vi "FIR Windowed Coefficients.vi"(0 "filter type":T2, 1 "high cutoff freq: fh":dbl=0.45 format="%0.2f", 2 "window parameter":dbl=nan, 5 "sampling freq: fs":dbl=1.0 format="%0.2f", 7 "taps":i32=25 min=1, 9 "window":T1 items=["Rectangle"=0, "Hanning"=1, "Hamming"=2, "Blackman-Harris"=3, "Exact Blackman"=4, "Blackman"=5, "Flat Top"=6, "4 Term B-Harris "=7, "7 Term B-Harris"=8, "Low Sidelobe"=9, "Blackman Nuttall"=11, "Triangle"=30, "Bartlett-Hanning"=31, "Bohman"=32, "Parzen"=33, "Welch"=34, "Kaiser"=60, "Dolph-Chebyshev"=61, "Gaussian"=62], 11 "option":enum32{"not scaled", "scaled"}(ring), 12 "low cutoff freq: fl":dbl=0.125 format="%0.2f") -> (4 "FIR Windowed Coefficients":dbl[](array[numeric]), 15 "error":i32)   [LabVIEW 2017, in "NI_AALBase.lvlib"]
doc: "Generates the set of filter coefficients you need to implement an FIR windowed filter."
uses:
  <vilib>/Analysis/NI_AALBase.lvlib
  <vilib>/Analysis/3filter.llb/Filter Passband Type.ctl
  <vilib>/Analysis/4window.llb/windowTd.ctl
  <vilib>/Analysis/1siggen.llb/Ramp Pattern by Samples.vi
  <vilib>/Analysis/4window.llb/Symmetric Window (DBL).vi
  <vilib>/Analysis/NI_AALPro.lvlib
panel:
  # "FIR Windowed Filter Coefficients"
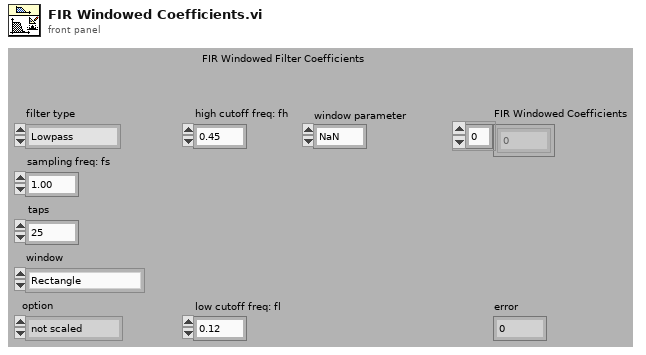
[diagram p1: front panel]
types:
  T1 = typedef "NI_AALPro.lvlib/windowTd.ctl" = u32
  T2 = typedef "NI_AALBase.lvlib/Filter Passband Type.ctl" = enum32{"Lowpass", "Highpass", "Bandpass", "Bandstop"}
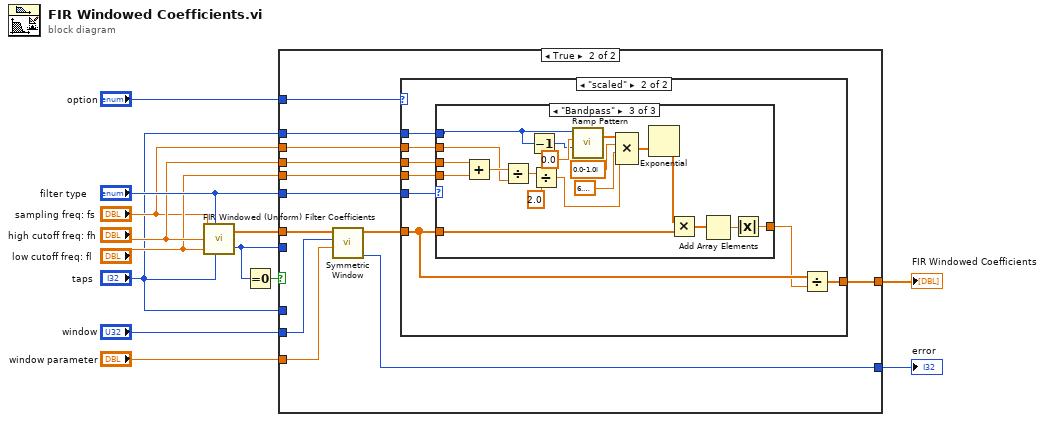
[diagram p0: block diagram]
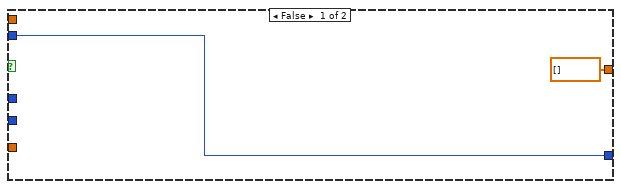
[diagram p2: hidden frame]
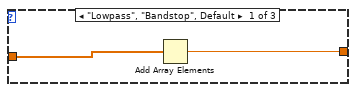
[diagram p4: hidden frame]
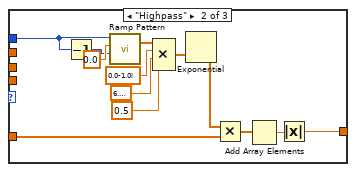
[diagram p5: hidden frame]
diagram:
  n1 = call <vilib>:"FIR Windowed (Uniform) Filter Coefficients.vi"("sampling freq: fs"="sampling freq: fs", "filter type"="filter type", "high cutoff freq: fh"="high cutoff freq: fh", "low cutoff freq: fl"="low cutoff freq: fl", "taps"="taps") -> ("FIR Coefficients"=w1:dbl[], "error"=w3:i32)
  n2 = Equal To 0?(x=w3) -> (x = 0?=w8:bool)
  n3 = case shown="True" w8 {
    tunnel: w1 -> [_ w18]
    tunnel: "filter type" -> [_ w27]
    tunnel: "high cutoff freq: fh" -> [_ w26]
    tunnel: "low cutoff freq: fl" -> [_ w25]
    tunnel: "sampling freq: fs" -> [_ w24]
    tunnel: [dbl[] [] w23] -> w9
    tunnel: "taps" -> [_ w22]
    tunnel: "window parameter" -> [_ w21]
    tunnel: "window" -> [_ w20]
    tunnel: "taps" -> [_ _]
    tunnel: "option" -> [_ w19]
    tunnel: w3 -> [w14 _]
    tunnel: [w14 w16] -> w2
    frame False {
    }
    frame True {
      n4 = call-poly <vilib>:"Symmetric Window.vi"("window parameter"=w21, "window"=w20, "X"=w18) -> ("error"=w16:i32, "Windowed X"=w17:dbl[])  [unwired: 7 out]
      n5 = case shown="\"scaled\"" w19 {
        tunnel: w27 -> [_ w36]
        tunnel: w22 -> [_ w35]
        tunnel: w26 -> [_ w34]
        tunnel: w25 -> [_ w33]
        tunnel: w24 -> [_ w32]
        tunnel: w17 -> [w28 w31]
        tunnel: [w28 w29] -> w23
        frame "not scaled", Default {
        }
        frame "scaled" {
          n6 = case shown="\"Bandpass\"" w36 {
            tunnel: w31 -> [w38 w45 w54]
            tunnel: [w37 w42 w52] -> w30
            tunnel: w35 -> [_ w40 w55]
            tunnel: w34 -> [_ _ w70]
            tunnel: w33 -> [_ _ w69]
            tunnel: w32 -> [_ _ w67]
            frame "Lowpass", "Bandstop", Default {
              n7 = Add Array Elements(numeric array=w38) -> (sum=w37:dbl)
            }
            frame "Highpass" {
              n8 = Decrement(x=w40) -> (x-1=w41:i32)
              n9 = call-poly <vilib>:"Ramp Pattern.vi"("start"=w41, "end"=0.0 ("start"), "samples"=w40) -> ("Ramp Pattern"=w50:dbl[])  [unwired: 7 in, 1 out]
              n10 = Compound Arithmetic op=MULTIPLY(w50, cdb 0.0-1.0i, 6.283185307179586, 0.5 ("start")) -> (w49:cdb[])
              n11 = Exponential(1:w49) -> (0:w46:cdb[])
              n12 = Multiply(x=w46, y=w45) -> (x*y=w44:cdb[])
              n13 = Add Array Elements(numeric array=w44) -> (sum=w43:cdb)
              n14 = Absolute Value(x=w43) -> (abs(x)=w42:dbl)
            }
            frame "Bandpass" {
              n15 = Add(x=w70, y=w69) -> (x+y=w68:dbl)
              n16 = Divide(x=w68, y=w67) -> (x/y=w66:dbl)
              n17 = Decrement(x=w55) -> (x-1=w56:i32)
              n18 = Divide(x=w66, y=2.0) -> (x/y=w53:dbl)
              n19 = call-poly <vilib>:"Ramp Pattern.vi"("start"=w56, "end"=0.0 ("start"), "samples"=w55) -> ("Ramp Pattern"=w63:dbl[])  [unwired: 7 in, 1 out]
              n20 = Compound Arithmetic op=MULTIPLY(w63, cdb 0.0-1.0i, 6.283185307179586, w53) -> (w62:cdb[])
              n21 = Exponential(1:w62) -> (0:w59:cdb[])
              n22 = Multiply(x=w59, y=w54) -> (x*y=w58:cdb[])
              n23 = Add Array Elements(numeric array=w58) -> (sum=w57:cdb)
              n24 = Absolute Value(x=w57) -> (abs(x)=w52:dbl)
            }
          }
          n25 = Divide(x=w31, y=w30) -> (x/y=w29:dbl[])
        }
      }
    }
  }
  "FIR Windowed Coefficients" <- w9
  "error" <- w2
